vi "溶解氧电极校准.vi"() -> ()   [LabVIEW 2016, in "斯坦道多参数.lvlib"]
uses:
  <vilib>/Utility/miscctls.llb/LVPointTypeDef.ctl
  <vilib>/Analysis/NI_AALBase.lvlib
panel:
  in  "盐度自动获取":bool
  out "滤波设定":dbl
  out "标液2":string="饱和标准液"
  out "标液1":string="零点标准液"
  in  "刷新按钮":bool
  out "第二点信号值":dbl
  out "第一点信号值":dbl
  out "通讯状态":string
  out "第二点校准值":dbl
  out "第一点校准值":dbl
  out "最小值":sgl format="%#.2f"
  out "最大值":sgl format="%#.2f"
  in  "校准模式":u16(ring)=1 items=["两点校准", "单点校准"]
  in  "校准停止":bool
  in  "校准启动":bool
  out "波形图表":sgl(graph) caption="历史曲线"
  out "变异系数":dbl format="%#.6f"
  out "standard deviation":dbl caption="标准差" format="%#.2f"
  out "mean":dbl caption="均值" format="%#.2f"
  out "测量读值":dbl caption="测量值" format="%#.2f"
  out "偏移值补偿":dbl caption="溶解氧偏移修正值" format="%#.2f"
  out "饱和度值":dbl format="%#.2f"
  out "提示":string
  out "气压补偿值":dbl format="%#.2f"
  out "盐度补偿值":dbl format="%#.2f"
  out "电极斜率":dbl format="%#.6f"
  out "电极零点":dbl format="%#.6f"
  # "溶解氧电极设定"
  # "%"
  # "%"
  # "ppt"
  # "hPa"
  # "请选择校准模式:"
  # "mg/L"
  # "%"
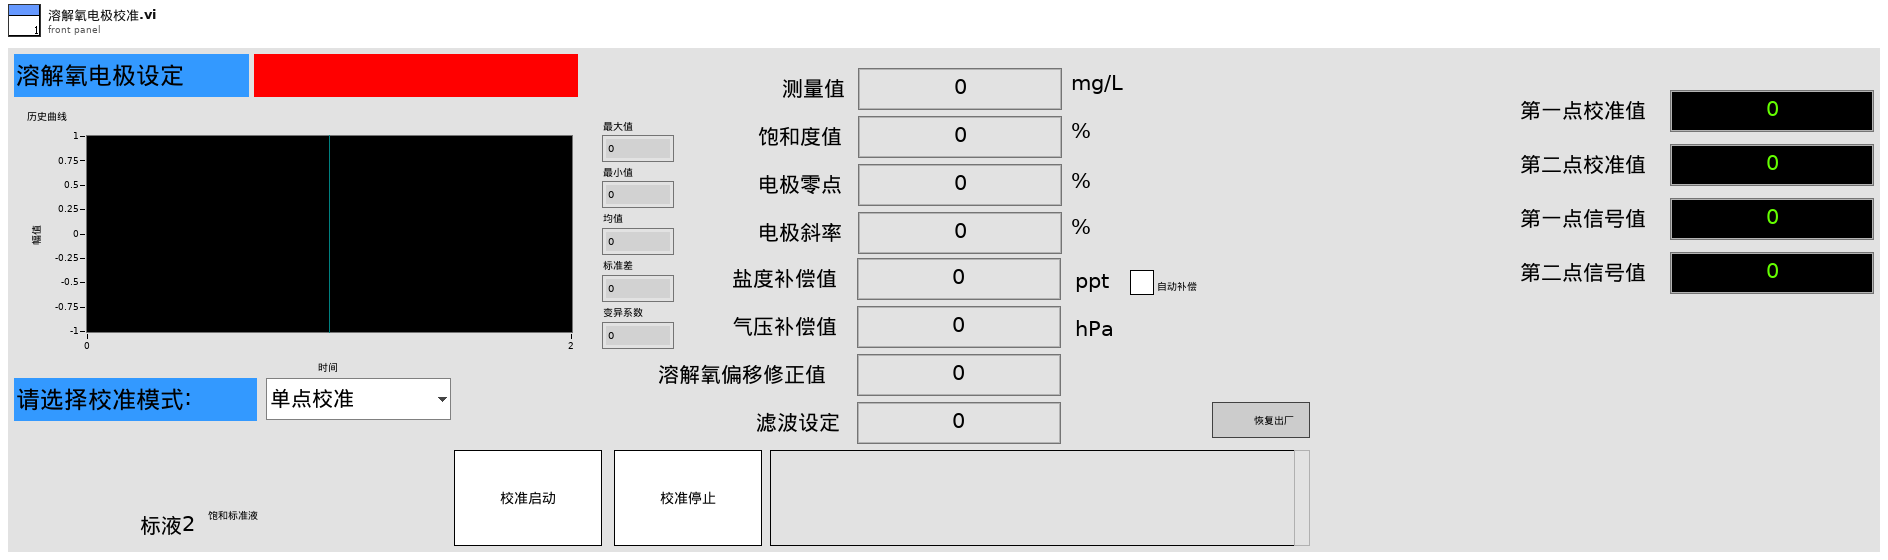
[diagram p1: front panel]
types:
  T1 = enum16{"pH", "DO", "Cond", "Turb", "ORP", "叶绿素a", "藻密度"}
  T2 = typedef "LVPointTypeDef.ctl" = cluster{"Horizontal":i16, "Vertical":i16}
  T3 = cluster{"电极状态标志":u16, "电极型号标志":u16, "溶解氧测量值":sgl, "温度测量值":sgl, "溶解氧饱和度值":sgl, "盐度补偿值":sgl, "大气压补偿值":sgl, "溶解氧偏移修正值":sgl, "温度偏移修正值":sgl, "手动温度补偿值":sgl, "溶解氧电极零点":sgl, "溶解氧电极斜率":sgl, "第1点标准值记录":sgl, "第1点信号值记录":sgl, "第1点温度值记录":sgl, "第2点标准值记录":sgl, "第2点信号值记录":sgl, "第2点温度值记录":sgl, "命令滤波设定":u16, "温度模式":enum16{"ATC", "MTC"}, "生产批次":u16, "电极序号":u16, "串口地址":u16, "串口波特率":enum16{"9600", "19200", "115200"}, "串口校验位":enum16{"NONE", "ODD", "EVEN"}, "串口停止位":enum16{"1bit", "2bit"}, "第一点标准值":sgl, "第二点标准值":sgl}
  T4 = enum8{"Enabled", "Disabled", "Disabled and Grayed Out"}
  T5 = cluster{"ph":bool, "DO":bool, "Cond":bool, "Turb":bool, "叶绿素a":bool, "藻密度":bool, "ORP":bool, "COD":bool}
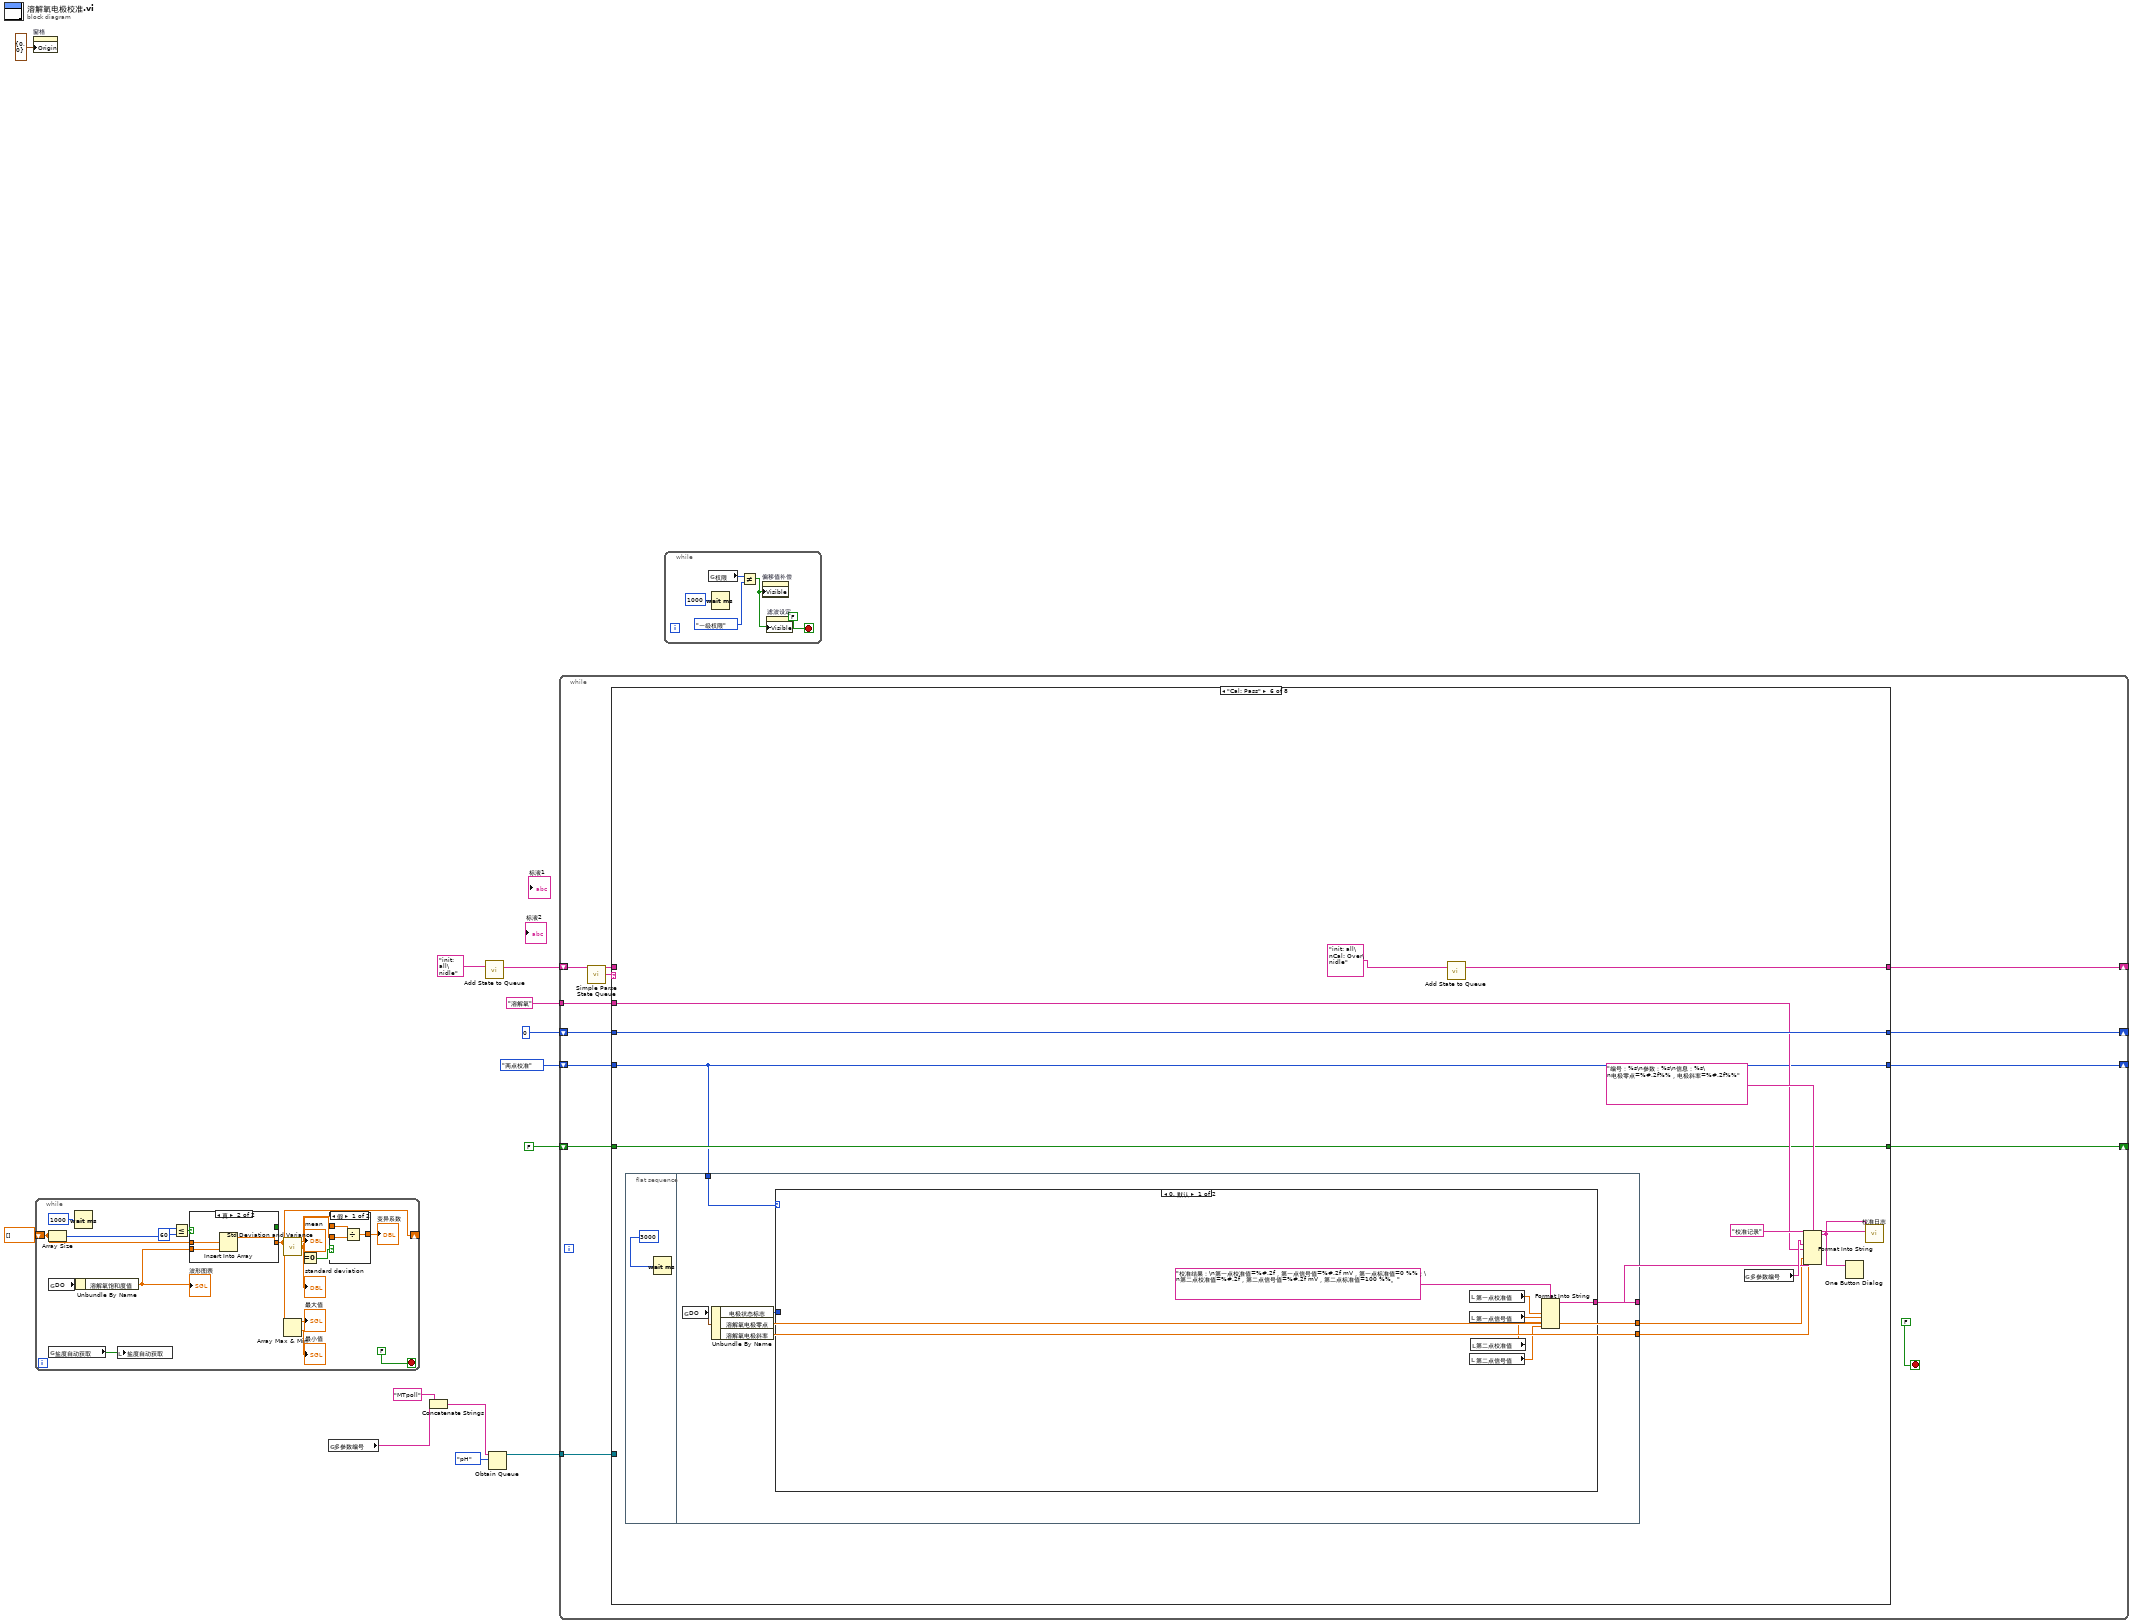
[diagram p0: block diagram]
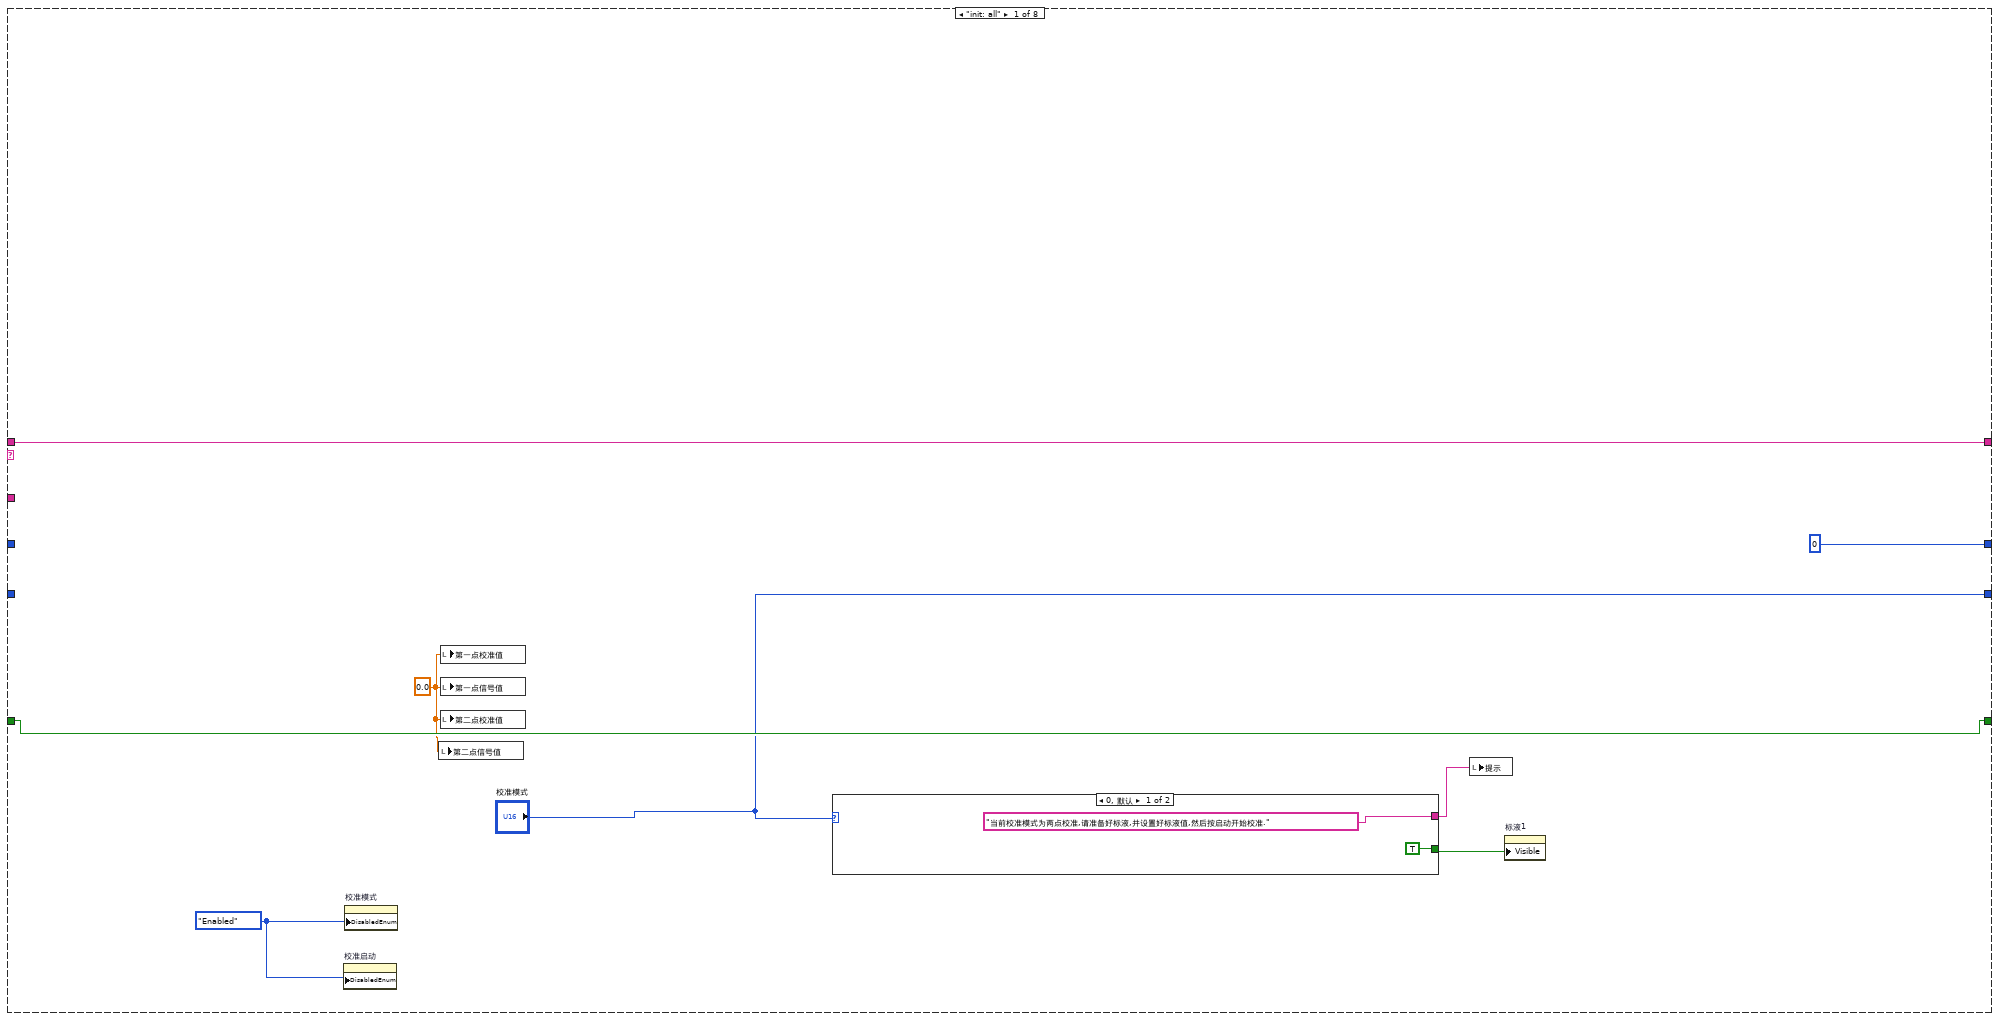
[diagram p2: hidden frame]
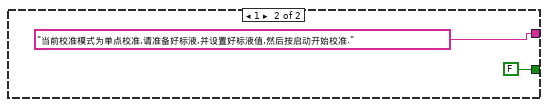
[diagram p3: hidden frame]
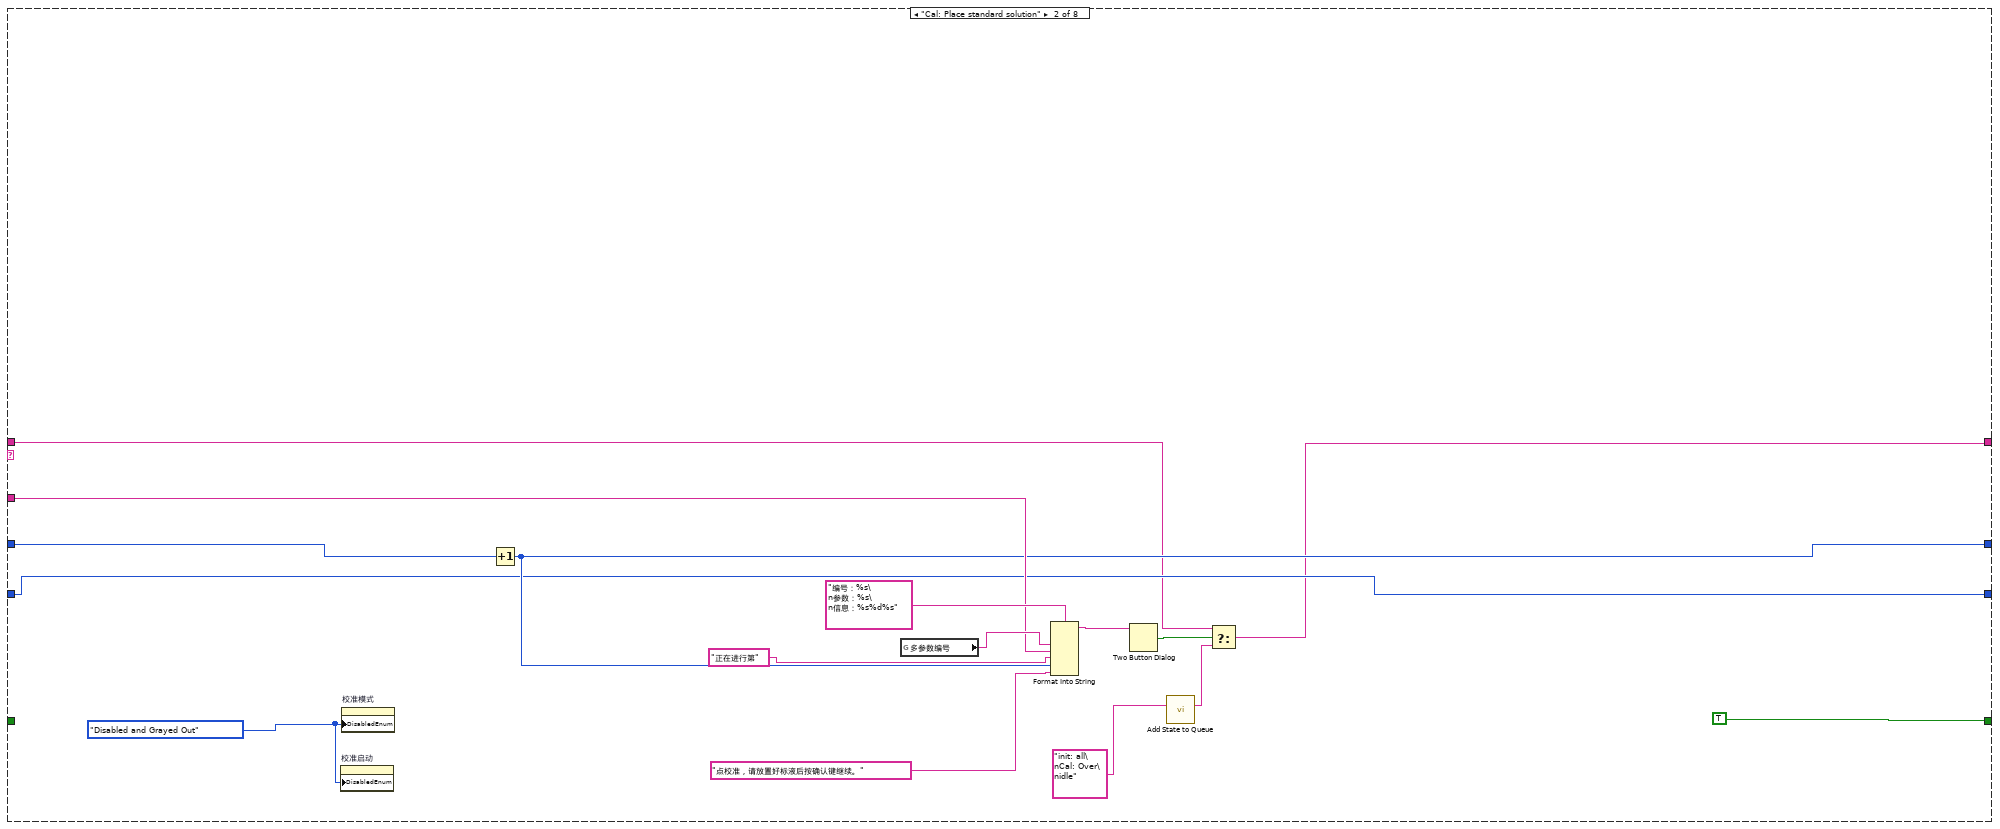
[diagram p4: hidden frame]
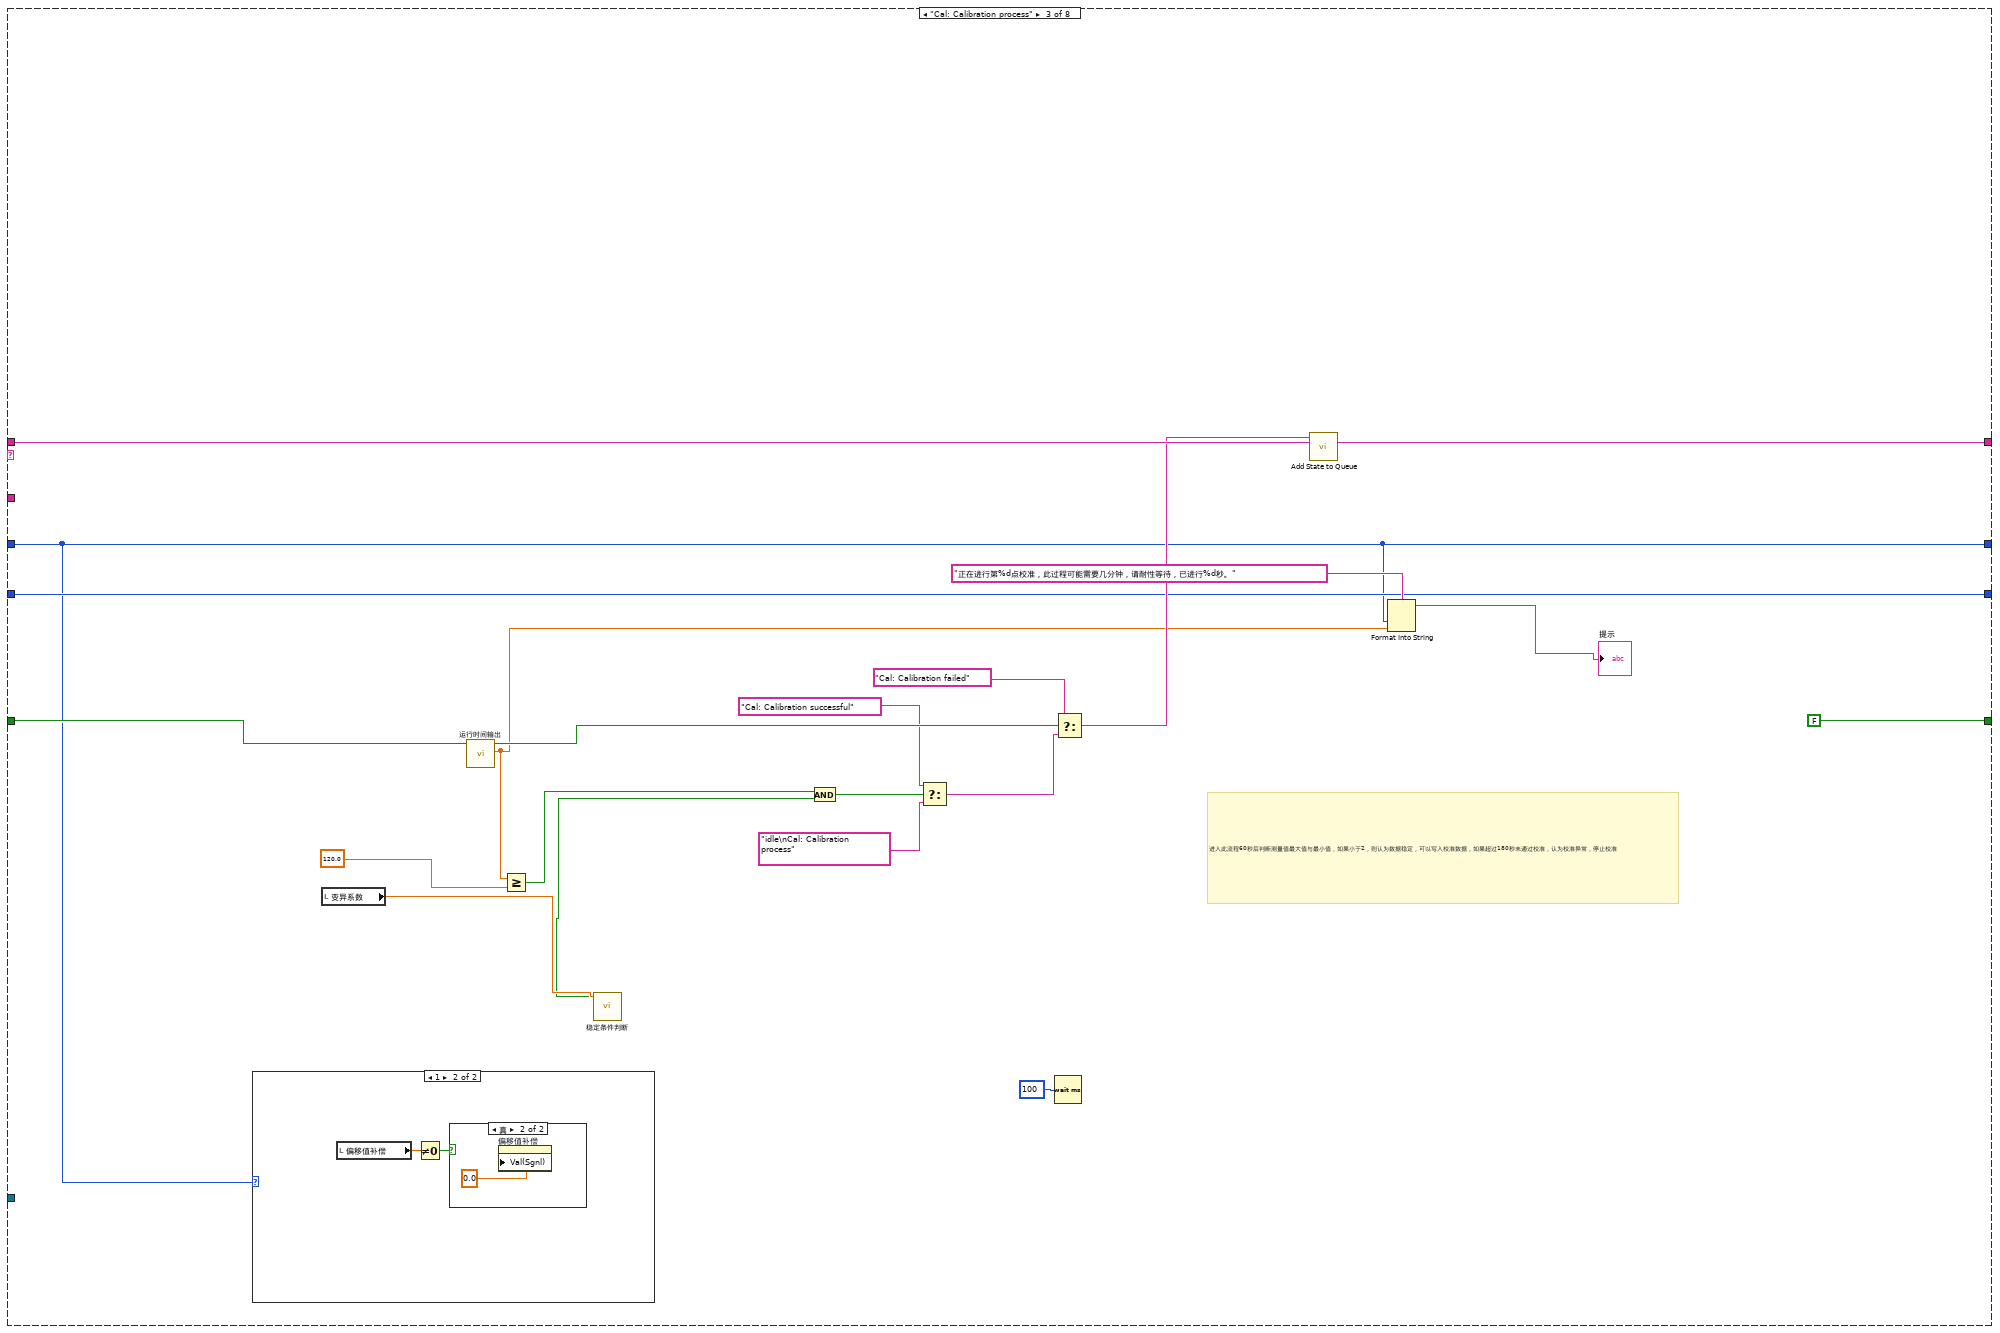
[diagram p5: hidden frame]
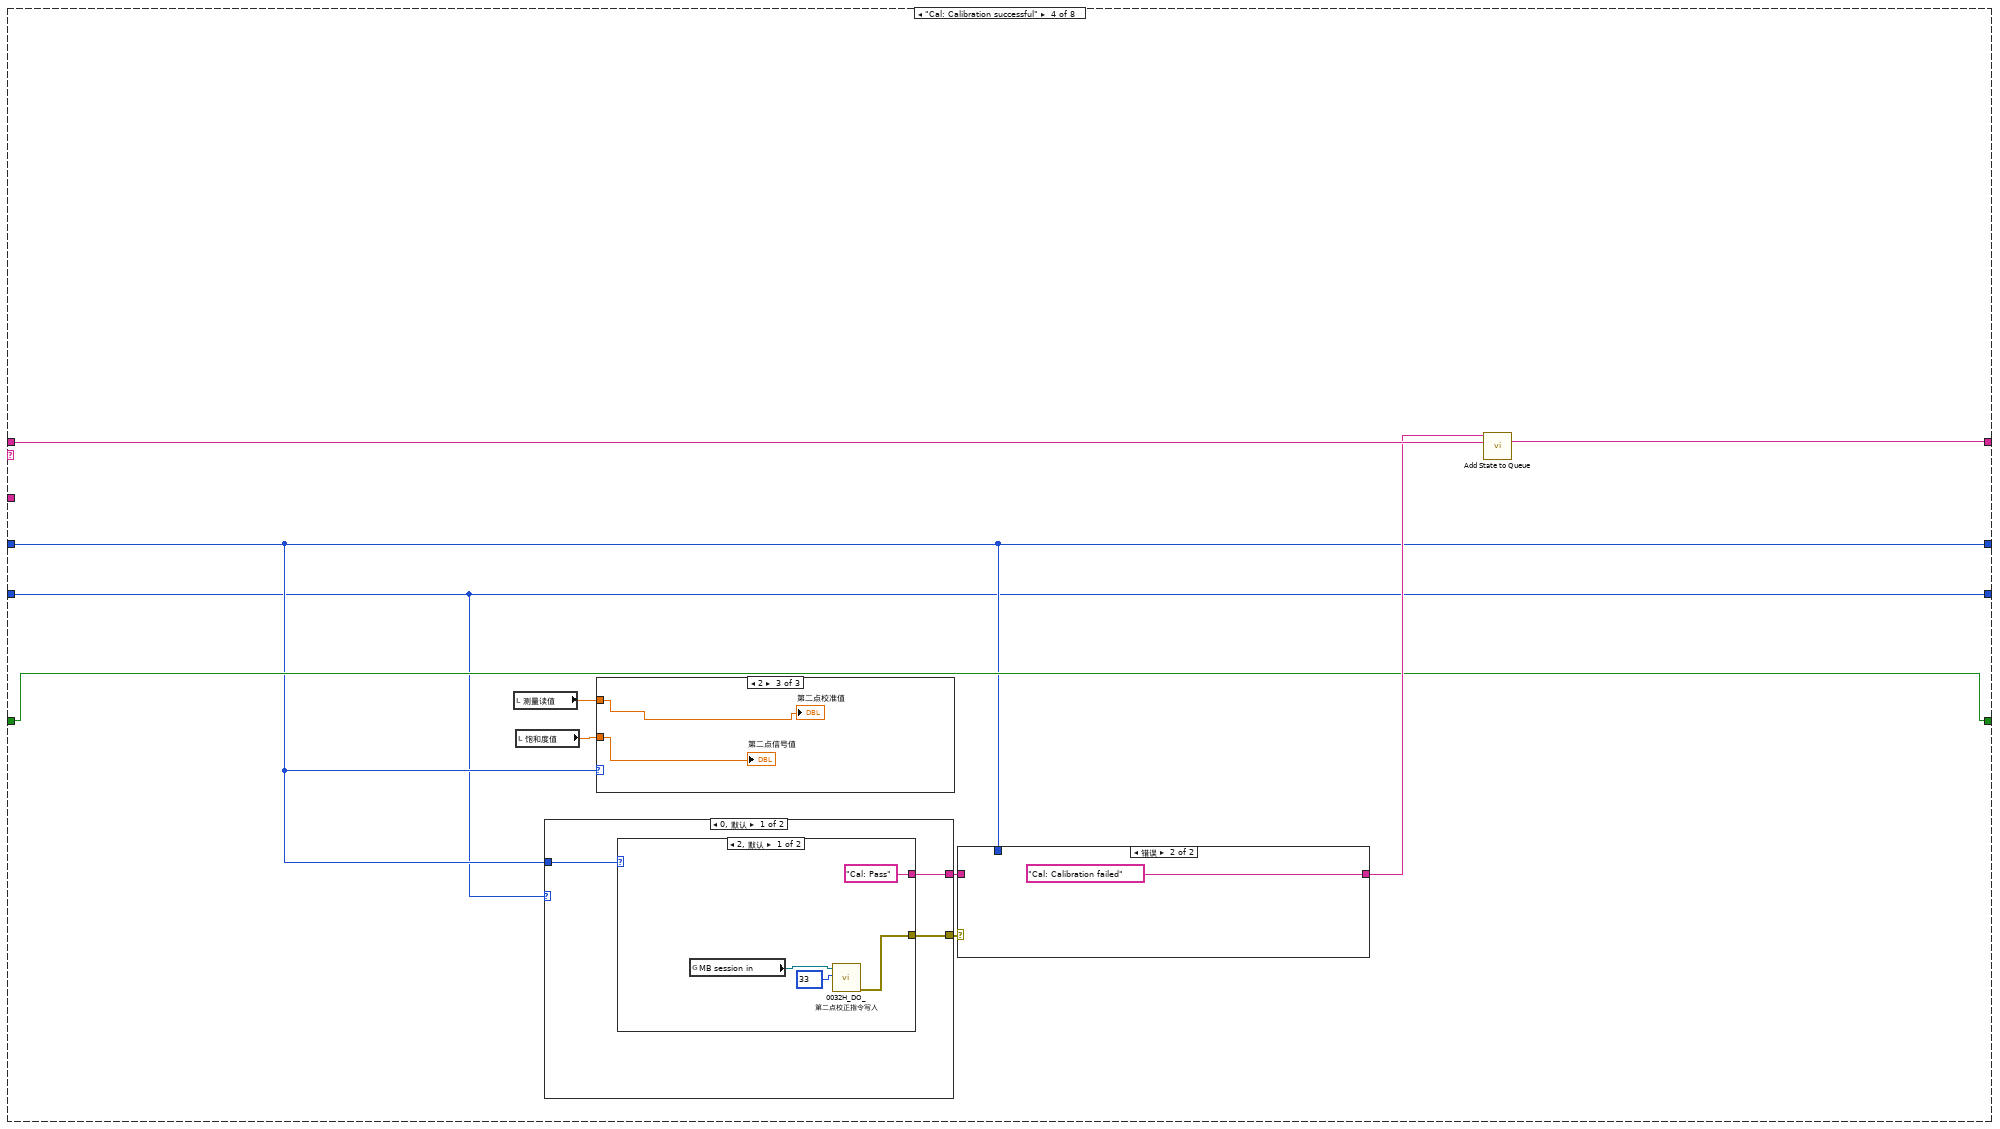
[diagram p8: hidden frame]
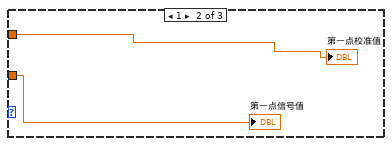
[diagram p10: hidden frame]
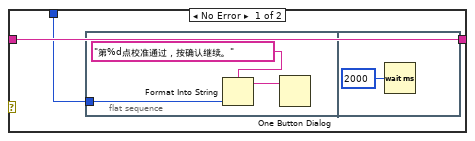
[diagram p11: hidden frame]
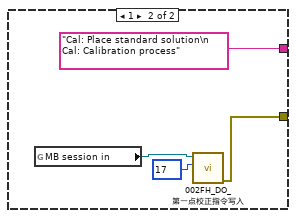
[diagram p12: hidden frame]
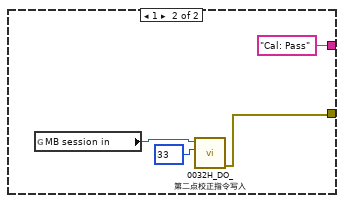
[diagram p13: hidden frame]
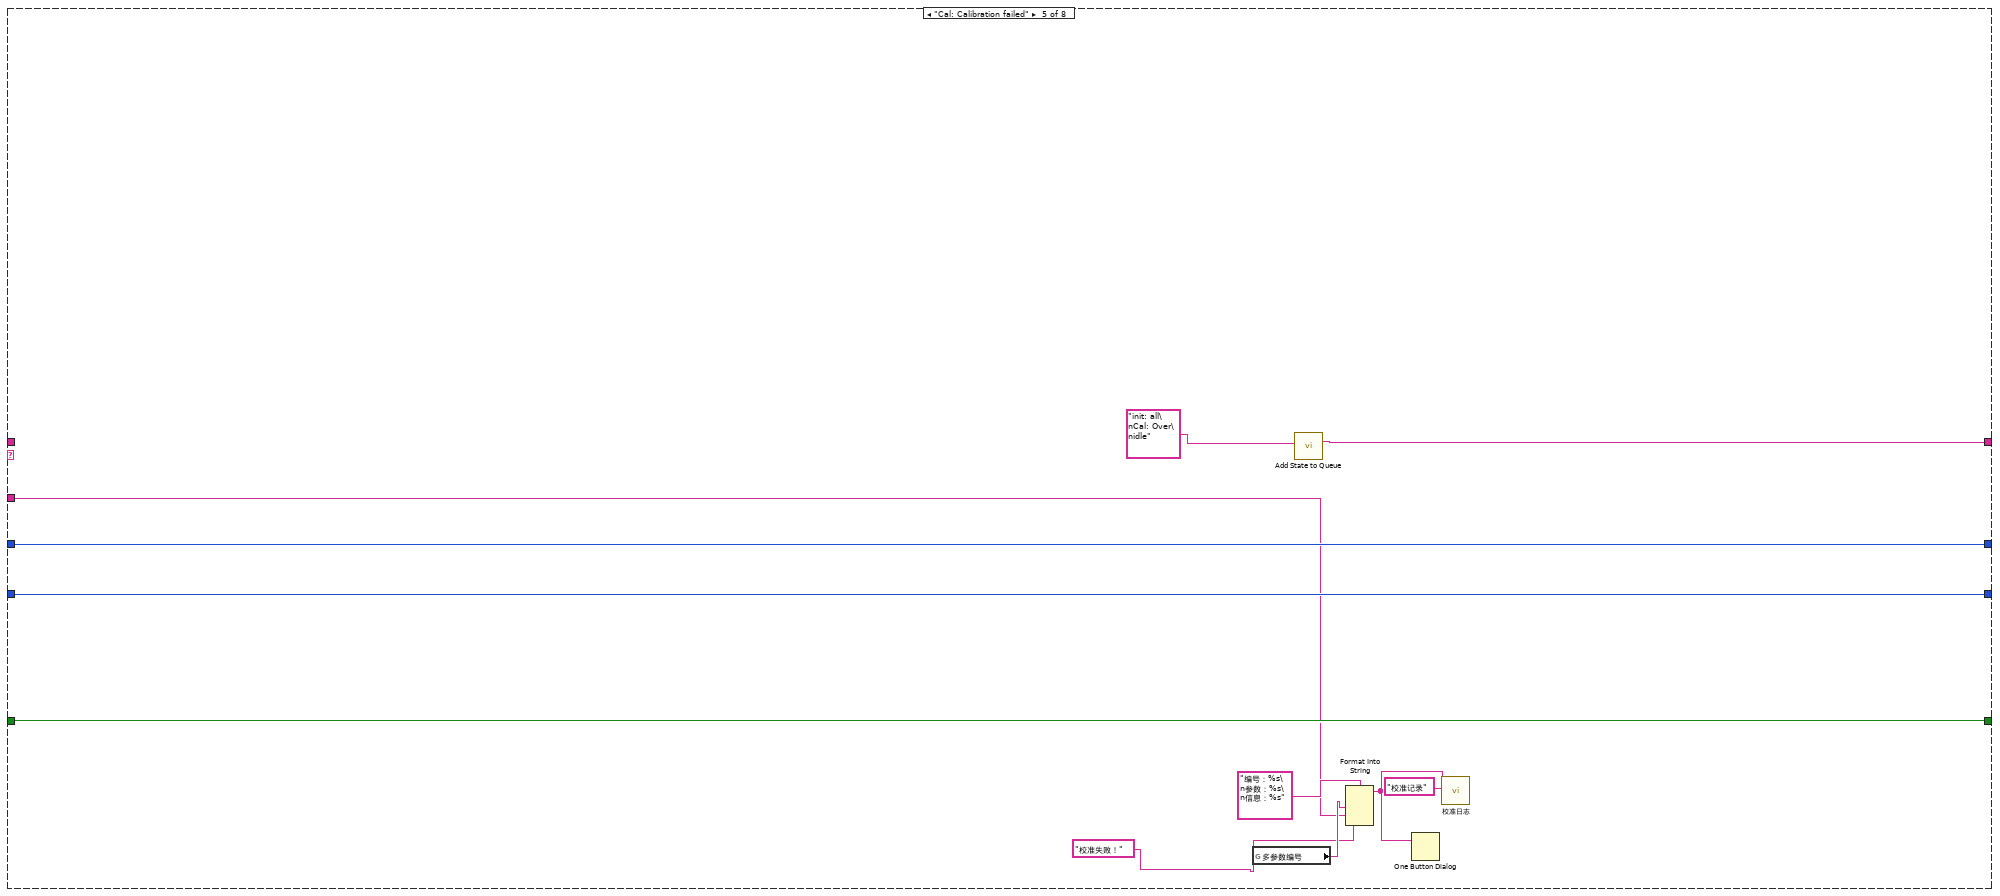
[diagram p14: hidden frame]
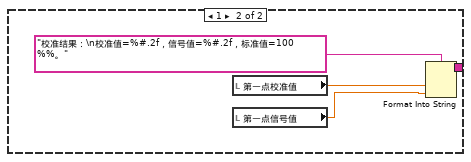
[diagram p15: hidden frame]
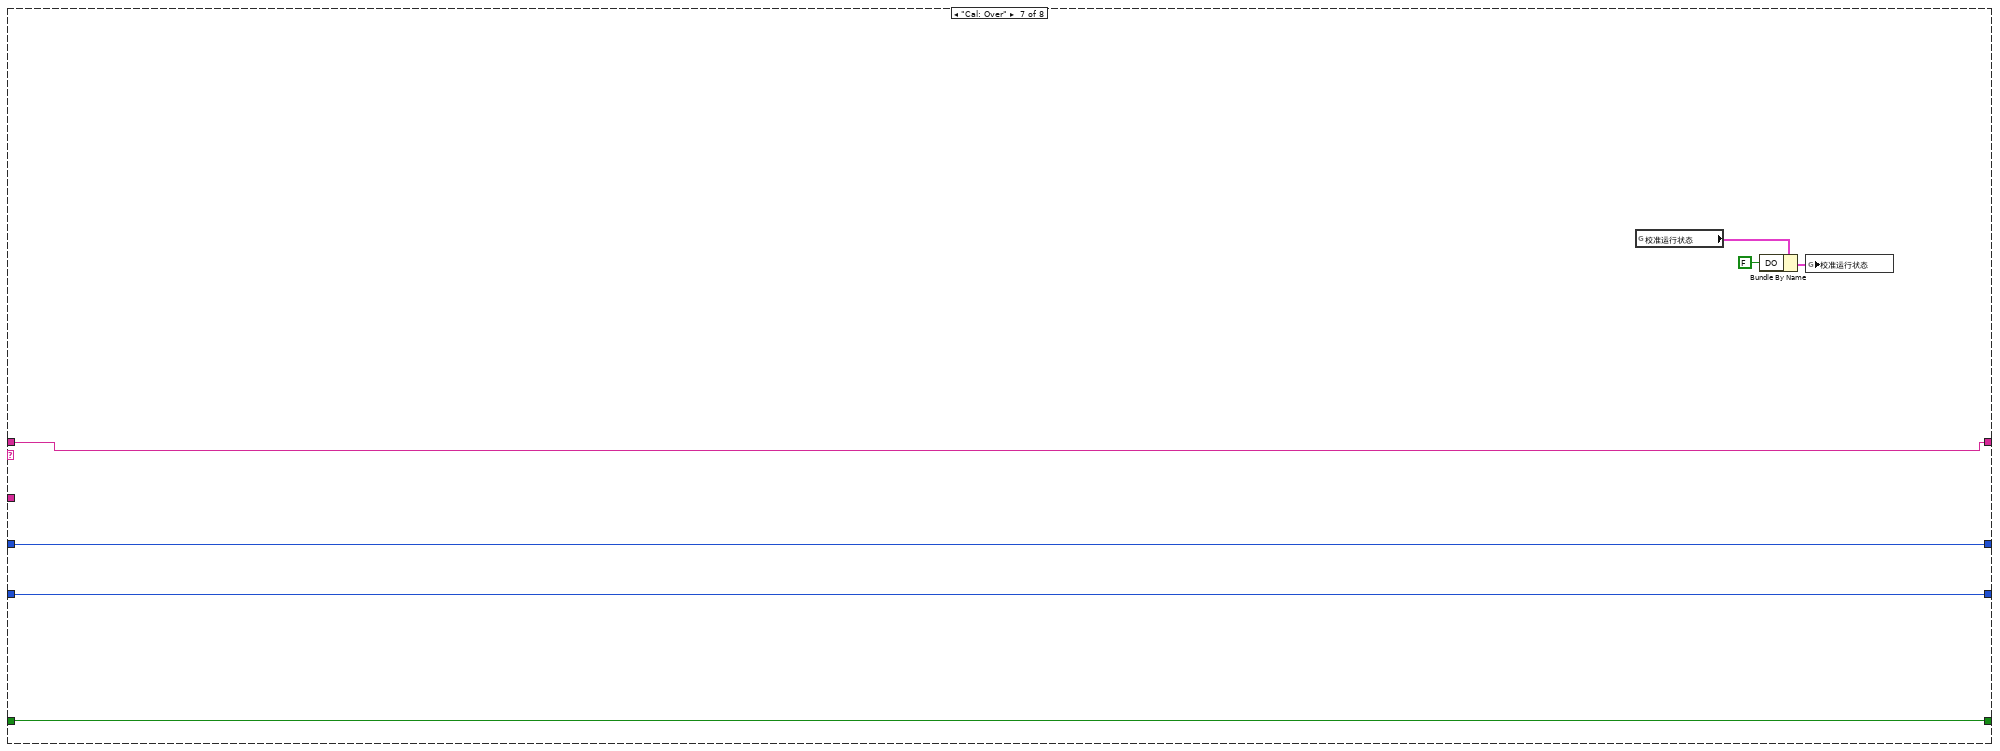
[diagram p16: hidden frame]
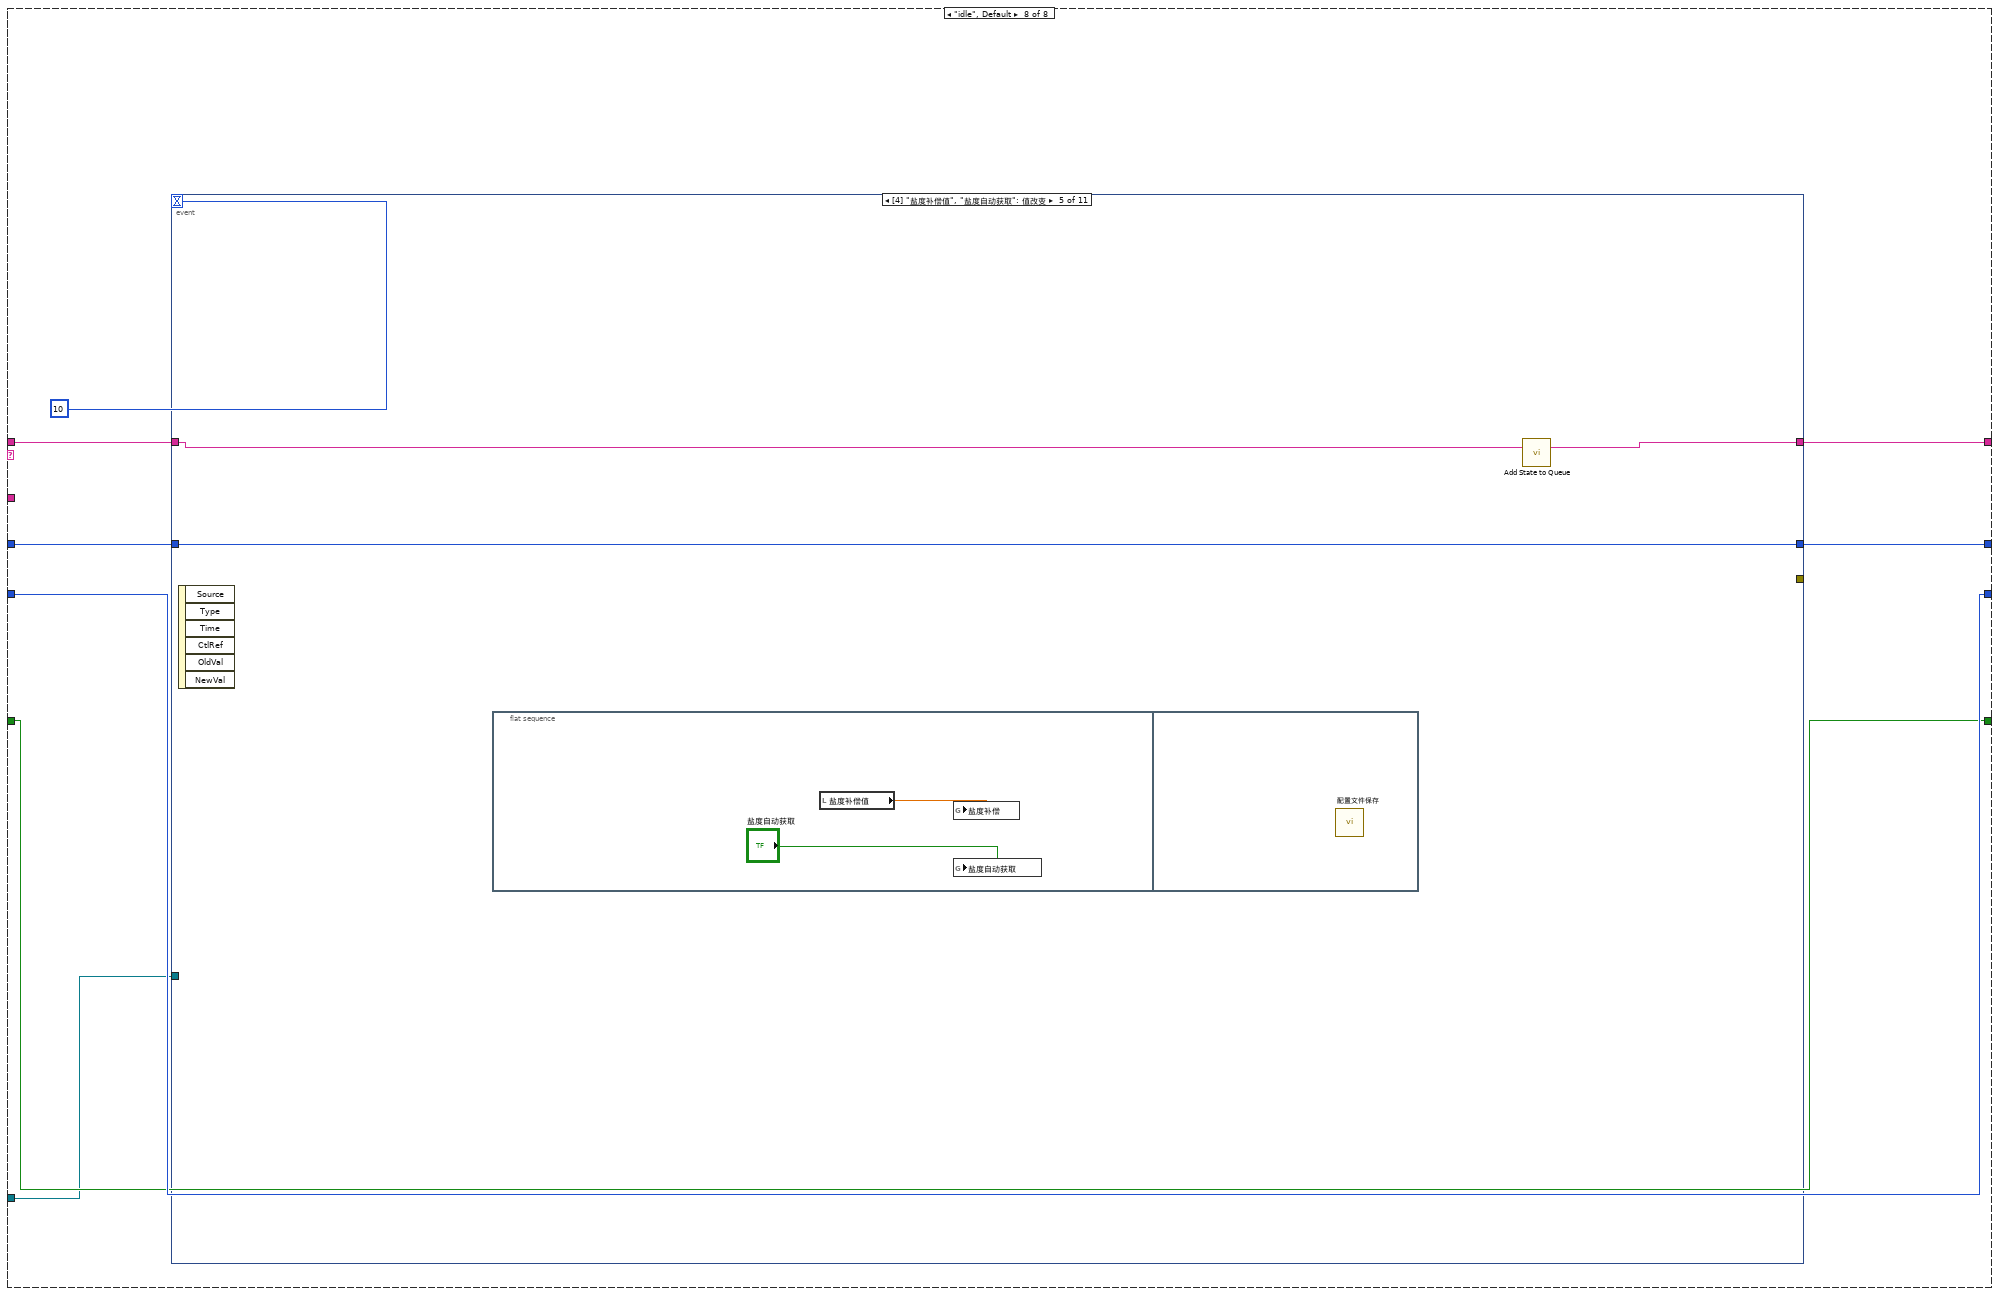
[diagram p17: hidden frame]
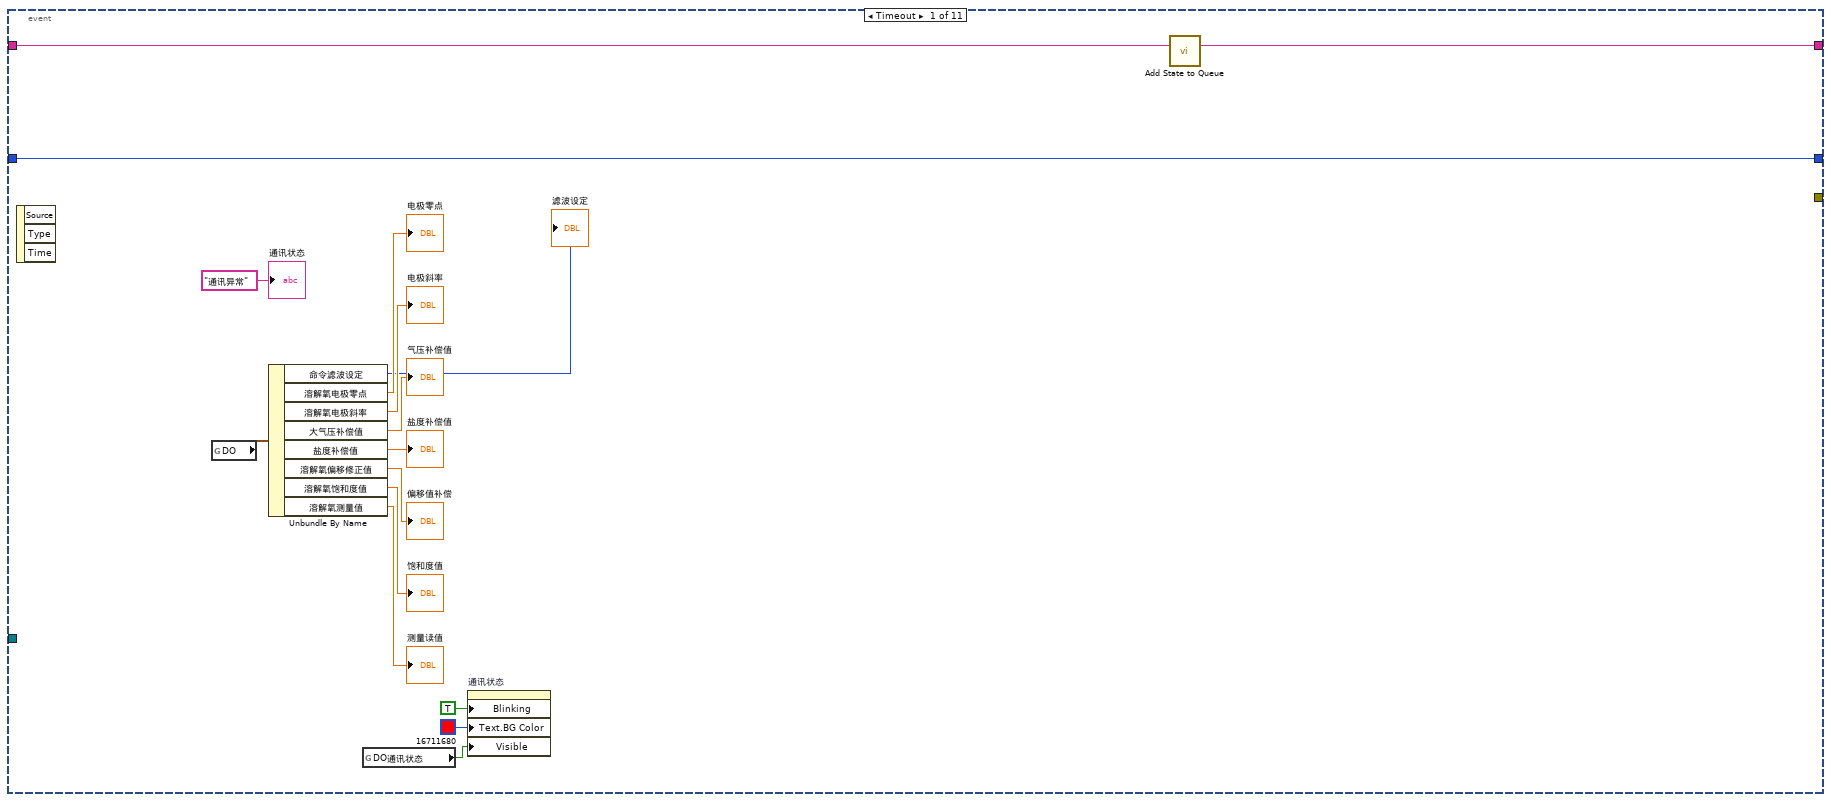
[diagram p18: hidden frame]
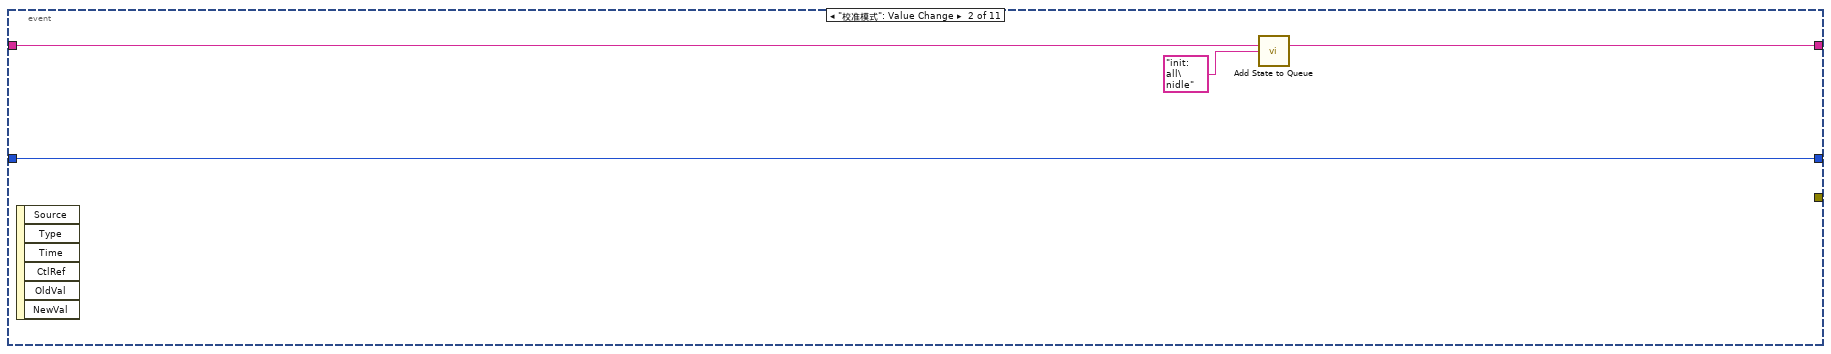
[diagram p19: hidden frame]
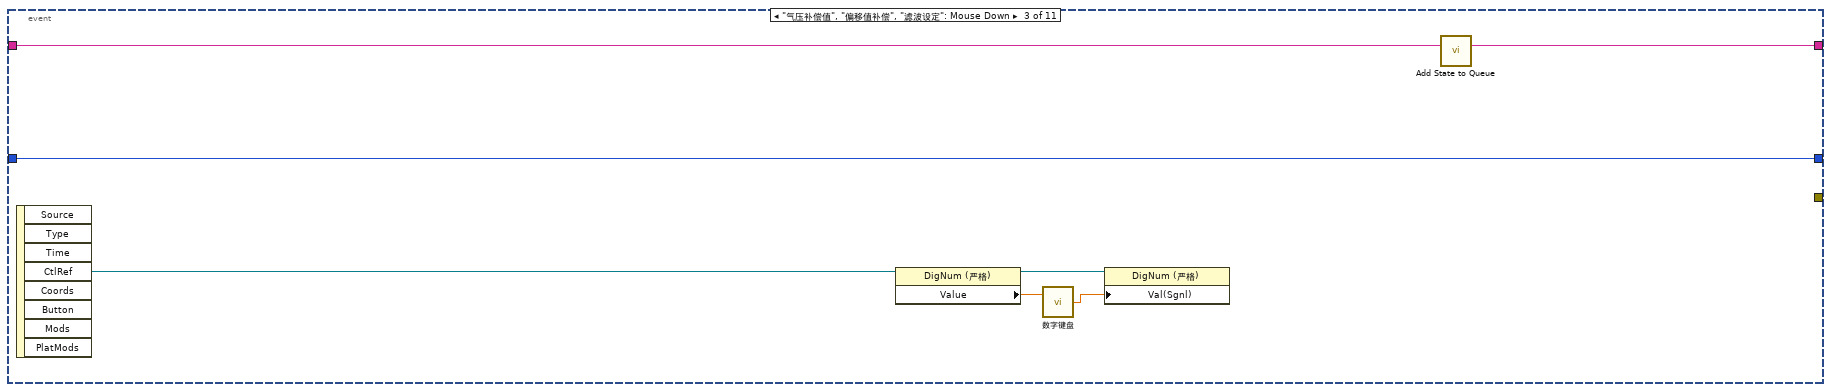
[diagram p20: hidden frame]
diagram:
  n1 = property on="窗格" class="Pane"("Origin"=T2 {"Horizontal"=0, "Vertical"=0} ("原点")) -> ()  [unwired: 2 in, 2 out]
  n2 = while {
    shift-right: [w18] -> _
    shift-left: sgl[] [] -> [w25]
    stop <- FALSE stop-if-true
    n3 = Array Size(array=w25) -> (size(s)=w27:i32)
    n4 = global read "国弘过程全局变量.vi" "DO"() -> (w21:T3)
    n5 = global read "断电保存变量.vi" "盐度自动获取"() -> (w14:bool)
    n6 = Wait (ms)(milliseconds to wait=u32 1000 ("等待时间（毫秒）")) -> ()  [unwired: 1 out]
    n7 = Unbundle By Name(w21) -> ("溶解氧饱和度值"=w15:sgl)
    "波形图表" <- w15
    n8 = local write "盐度自动获取"(w14) -> ()
    n9 = Less Or Equal?(x=w27, y=60) -> (x <= y?=w26:bool)
    n10 = case shown="真" w26 {
      tunnel: w25 -> [w38 w41]
      tunnel: w15 -> [w36 w40]
      tunnel: [w34 w39] -> w18
      tunnel: [TRUE _] -> _
      frame False {
        n11 = Replace Array Subset(array=w38, new element=w36) -> (w37:sgl[])  [unwired: 1 in]
        n12 = Rotate 1D Array(1:w37, 2:-1 ("n")) -> (0:w34:sgl[])
      }
      frame True {
        n13 = Insert Into Array(array=w41, new element=w40) -> (w39:sgl[])  [unwired: 1 in]
      }
    }
    n14 = call <vilib>:"Std Deviation and Variance.vi"("X"=w18) -> ("mean"=w20:dbl, "standard deviation"=w19:dbl)  [unwired: 1 in, 1 out]
    "mean" <- w20
    "standard deviation" <- w19
    n15 = Array Max & Min(array=w18) -> (max value=→"最大值":sgl, min value=→"最小值":sgl)  [unwired: 2 out]
    n16 = Equal To 0?(x=w20) -> (x = 0?=w24:bool)
    n17 = case shown="假" w24 {
      tunnel: w19 -> [w32 _]
      tunnel: [w31 _] -> w23
      tunnel: w20 -> [w30 _]
      frame False {
        n18 = Divide(x=w32, y=w30) -> (x/y=w31:dbl)
      }
      frame True {
      }
    }
    "变异系数" <- w23
  }
  n19 = global read "多参数全局变量.vi" "多参数编号"() -> (w2:string)
  n20 = Concatenate Strings("MTpoll" ("名称（未命名）"), w2) -> (w4:string)
  n21 = call "Add State to Queue.vi"("State(s) In (\"\")"="init: all\nidle" ("State(s) In (\"\")")) -> ("States Out"=w10:string)  [unwired: 14 in]
  n22 = Obtain Queue(name (unnamed)=w4, element data type=T1."pH" ("枚举")) -> (queue out=w1:refnum<queue>)  [unwired: 3 in, 2 out]
  n23 = while {
    shift-right: [w50] -> _
    shift-left: w10 -> [w54]
    shift-right: [w47] -> _
    shift-left: 0 -> [w49]
    tunnel: "溶解氧" ("State(s) In (\"\")") -> [w48]
    shift-right: [w45] -> _
    shift-left: enum16{"两点校准", "单点校准"}."两点校准" ("校准模式") -> [w46]
    shift-right: [w43] -> _
    shift-left: FALSE -> [w44]
    tunnel: w1 -> [w42]
    stop <- FALSE stop-if-true
    n24 = call "Simple Parse State Queue.vi"("State Queue"=w54) -> ("Remain States"=w51:string, "Next State"=w52:string)  [unwired: 13 in]
    n25 = case shown="\"Cal: Pass\"" w52 {
      tunnel: w51 -> [w62 w70 w102 w114 _ _ w190 w198]
      tunnel: [w62 w69 w101 w113 w150 w157 w190 w197] -> w50
      tunnel: w49 -> [_ w78 w87 w108 w153 w166 w189 w195]
      tunnel: w48 -> [_ w79 _ _ w144 w162 _ _]
      tunnel: [0 w76 w87 w108 w153 w166 w189 w196] -> w47
      tunnel: w46 -> [_ w75 w88 w107 w152 w158 w188 w194]
      tunnel: ["校准模式" w75 w88 w107 w152 w158 w188 w194] -> w45
      tunnel: w44 -> [w59 _ w90 w109 w151 w161 w187 w192]
      tunnel: [w59 TRUE FALSE w109 w151 w161 w187 w192] -> w43
      tunnel: w42 -> [_ _ _ _ _ _ _ w191]
      frame "init: all" {
        w57 = T4."Enabled" ("禁用")
        w58 = 0.0 ("第一点校准值")
        n26 = property on="校准启动" class="Bool"("DisabledEnum"=w57) -> ()  [unwired: 2 in, 2 out]
        n27 = property on="校准模式" class="Ring (严格)"("DisabledEnum"=w57) -> ()  [unwired: 2 in, 2 out]
        n28 = local write "第二点信号值"(w58) -> ()
        n29 = local write "第一点校准值"(w58) -> ()
        n30 = local write "第一点信号值"(w58) -> ()
        n31 = local write "第二点校准值"(w58) -> ()
        n32 = case shown="0, 默认" "校准模式" {
          tunnel: ["当前校准模式为两点校准,请准备好标液,并设置好标液值,然后按启动开始校准." ("提示") "当前校准模式为单点校准,请准备好标液,并设置好标液值,然后按启动开始校准." ("提示")] -> w61
          tunnel: [TRUE ("可见") FALSE ("可见")] -> w55
          frame 0, Default {
          }
          frame 1 {
          }
        }
        n33 = local write "提示"(w61) -> ()
        n34 = property on="标液1" class="Str"("Visible"=w55) -> ()  [unwired: 2 in, 2 out]
      }
      frame "Cal: Place standard solution" {
        w68 = T4."Disabled and Grayed Out" ("禁用")
        n35 = property on="校准启动" class="Bool"("DisabledEnum"=w68) -> ()  [unwired: 2 in, 2 out]
        n36 = property on="校准模式" class="Ring (严格)"("DisabledEnum"=w68) -> ()  [unwired: 2 in, 2 out]
        n37 = Increment(x=w78) -> (x+1=w76:i32)
        n38 = global read "多参数全局变量.vi" "多参数编号"() -> (w81:string)
        n39 = Format Into String(format string="编号：%s\n参数：%s\n信息：%s%d%s" ("格式字符串"), w81, w79, "正在进行第" ("消息"), w76, "点校准，请放置好标液后按确认键继续。" ("消息")) -> (resulting string=w73:string)  [unwired: 2 in, 1 out]
        n40 = Two Button Dialog(message=w73) -> (T button?=w72:bool)  [unwired: 2 in]
        n41 = call "Add State to Queue.vi"("State(s) In (\"\")"="init: all\nCal: Over\nidle" ("State(s) In (\"\")")) -> ("States Out"=w71:string)  [unwired: 14 in]
        n42 = Select(t=w70, s=w72, f=w71) -> (s? t:f=w69:string)
      }
      frame "Cal: Calibration process" {
        # "进入此流程60秒后判断测量值最大值与最小值，如果小于2，则认为数据稳定，可以写入校准数据，如果超过180秒未通过校准，认为校准异常，停止校准"
        n43 = case shown="1" w87 {
          frame 0, Default {
          }
          frame 1 {
            n44 = local read "偏移值补偿"() -> (w104:dbl)
            n45 = Not Equal To 0?(x=w104) -> (x != 0?=w105:bool)
            n46 = case shown="真" w105 {
              frame False {
              }
              frame True {
                n47 = property on="偏移值补偿" class="DigNum (严格)"("Val(Sgnl)"=0.0 ("值(信号)")) -> ()  [unwired: 2 in, 2 out]
              }
            }
          }
        }
        n48 = local read "变异系数"() -> (w84:dbl)
        n49 = call "运行时间输出.vi"("初始化"=w90) -> ("Elapsed Time (s)"=w86:dbl, "Time has Elapsed"=w103:bool)  [unwired: 9 in]
        n50 = Greater Or Equal?(x=w86, y=120.0) -> (x >= y?=w98:bool)
        n51 = call "稳定条件判断.vi"("变异系数"=w84) -> ("布尔"=w83:bool)  [unwired: 10 in]
        n52 = And(x=w98, y=w83) -> (x .and. y?=w95:bool)
        n53 = Select(t="Cal: Calibration successful" ("State(s) In (\"\")"), s=w95, f="idle\nCal: Calibration process" ("State(s) In (\"\")")) -> (s? t:f=w94:string)
        n54 = Wait (ms)(milliseconds to wait=u32 100 ("等待时间（毫秒）")) -> ()  [unwired: 1 out]
        n55 = Select(t="Cal: Calibration failed" ("State(s) In (\"\")"), s=w103, f=w94) -> (s? t:f=w93:string)
        n56 = call "Add State to Queue.vi"("State(s) In Front (\"\")"=w93, "State(s) In (\"\")"=w102) -> ("States Out"=w101:string)  [unwired: 13 in]
        n57 = Format Into String(format string="正在进行第%d点校准，此过程可能需要几分钟，请耐性等待，已进行%d秒。" ("格式字符串"), w87, w86) -> (resulting string=→"提示":string)  [unwired: 2 in, 1 out]
      }
      frame "Cal: Calibration successful" {
        n58 = local read "测量读值"() -> (w110:dbl)
        n59 = local read "饱和度值"() -> (w111:dbl)
        n60 = case shown="0, 默认" w107 {
          tunnel: [w130 w139] -> w116
          tunnel: [w129 "Cal: Pass" ("State(s) In (\"\")")] -> w115
          tunnel: w108 -> [w128 _]
          frame 0, Default {
            n61 = case shown="2, 默认" w128 {
              tunnel: [w131 w135] -> w130
              tunnel: ["Cal: Pass" ("State(s) In (\"\")") "Cal: Place standard solution\n Cal: Calibration process" ("State(s) In (\"\")")] -> w129
              frame 2, Default {
                n62 = global read "多参数全局变量.vi" "MB session in"() -> (w132:refnum<class "MB_Master.lvclass">)
                n63 = call "0032H_DO_第二点校正指令写入.vi"("数值"=u16 33, "MB session in"=w132) -> ("error out"=w131:errorcluster)  [unwired: 8 in, 1 out]
              }
              frame 1 {
                n64 = global read "多参数全局变量.vi" "MB session in"() -> (w136:refnum<class "MB_Master.lvclass">)
                n65 = call "002FH_DO_第一点校正指令写入.vi"("数值"=u16 17, "MB session in"=w136) -> ("error out"=w135:errorcluster)  [unwired: 8 in, 1 out]
              }
            }
          }
          frame 1 {
            n66 = global read "多参数全局变量.vi" "MB session in"() -> (w141:refnum<class "MB_Master.lvclass">)
            n67 = call "0032H_DO_第二点校正指令写入.vi"("数值"=u16 33, "MB session in"=w141) -> ("error out"=w139:errorcluster)  [unwired: 8 in, 1 out]
          }
        }
        n68 = case shown="2" w108 {
          tunnel: w111 -> [_ w118 w120]
          tunnel: w110 -> [_ w117 w119]
          frame 0, Default {
          }
          frame 1 {
            "第一点信号值" <- w118
            "第一点校准值" <- w117
          }
          frame 2 {
            "第二点信号值" <- w120
            "第二点校准值" <- w119
          }
        }
        n69 = case shown="错误" w116 {
          tunnel: w115 -> [w122 _]
          tunnel: [w122 "Cal: Calibration failed" ("State(s) In (\"\")")] -> w112
          tunnel: w108 -> [w121 _]
          frame No Error {
            n70 = flat-sequence {
              tunnel: w121 -> [w123]
              frame #0 {
                n71 = Format Into String(format string="第%d点校准通过，按确认继续。" ("格式字符串"), w123) -> (resulting string=w125:string)  [unwired: 2 in, 1 out]
                n72 = One Button Dialog(message=w125) -> ()  [unwired: 1 in, 1 out]
              }
              frame #1 {
                n73 = Wait (ms)(milliseconds to wait=u32 2000 ("等待时间（毫秒）")) -> ()  [unwired: 1 out]
              }
            }
          }
          frame Error {
          }
        }
        n74 = call "Add State to Queue.vi"("State(s) In Front (\"\")"=w112, "State(s) In (\"\")"=w114) -> ("States Out"=w113:string)  [unwired: 13 in]
      }
      frame "Cal: Calibration failed" {
        n75 = global read "多参数全局变量.vi" "多参数编号"() -> (w147:string)
        n76 = call "Add State to Queue.vi"("State(s) In (\"\")"="init: all\nCal: Over\nidle" ("State(s) In (\"\")")) -> ("States Out"=w150:string)  [unwired: 14 in]
        n77 = Format Into String(format string="编号：%s\n参数：%s\n信息：%s" ("格式字符串"), w147, w144, "校准失败！" ("消息")) -> (resulting string=w146:string)  [unwired: 2 in, 1 out]
        n78 = One Button Dialog(message=w146) -> ()  [unwired: 1 in, 1 out]
        n79 = call "校准日志.vi"("table"="校准记录", "日志信息"=w146) -> ()  [unwired: 9 in, 1 out]
      }
      frame "Cal: Pass" {
        n80 = flat-sequence {
          tunnel: [w171] -> w159
          tunnel: w158 -> [w170]
          tunnel: [w169] -> w156
          tunnel: [w168] -> w155
          frame #0 {
            n81 = Wait (ms)(milliseconds to wait=u32 3000 ("等待时间（毫秒）")) -> ()  [unwired: 1 out]
          }
          frame #1 {
            n82 = global read "国弘过程全局变量.vi" "DO"() -> (w172:T3)
            n83 = Unbundle By Name(w172) -> ("电极状态标志"=w173:u16, "溶解氧电极零点"=w169:sgl, "溶解氧电极斜率"=w168:sgl)
            n84 = case shown="0, 默认" w170 {
              tunnel: [w179 w183] -> w171
              tunnel: w173 -> [_ _]
              frame 0, Default {
                n85 = local read "第一点校准值"() -> (w177:dbl)
                n86 = local read "第一点信号值"() -> (w178:dbl)
                n87 = local read "第二点信号值"() -> (w174:dbl)
                n88 = local read "第二点校准值"() -> (w175:dbl)
                n89 = Format Into String(format string="校准结果：\n第一点校准值=%#.2f，第一点信号值=%#.2f mV，第一点标准值=0 %%；\n第二点校准值=%#.2f，第二点信号值=%#.2f mV，第二点标准值=100 %%。" ("提示"), w177, w178, w175, w174) -> (resulting string=w179:string)  [unwired: 2 in, 1 out]
              }
              frame 1 {
                n90 = local read "第一点校准值"() -> (w182:dbl)
                n91 = local read "第一点信号值"() -> (w180:dbl)
                n92 = Format Into String(format string="校准结果：\n校准值=%#.2f，信号值=%#.2f，标准值=100 %%。" ("提示"), w182, w180) -> (resulting string=w183:string)  [unwired: 2 in, 1 out]
              }
            }
          }
        }
        n93 = call "Add State to Queue.vi"("State(s) In (\"\")"="init: all\nCal: Over\nidle" ("State(s) In (\"\")")) -> ("States Out"=w157:string)  [unwired: 14 in]
        n94 = global read "多参数全局变量.vi" "多参数编号"() -> (w163:string)
        n95 = Format Into String(format string="编号：%s\n参数：%s\n信息：%s\n电极零点=%#.2f%%，电极斜率=%#.2f%%" ("格式字符串"), w163, w162, w159, w156, w155) -> (resulting string=w160:string)  [unwired: 2 in, 1 out]
        n96 = One Button Dialog(message=w160) -> ()  [unwired: 1 in, 1 out]
        n97 = call "校准日志.vi"("table"="校准记录", "日志信息"=w160) -> ()  [unwired: 9 in, 1 out]
      }
      frame "Cal: Over" {
        n98 = global read "多参数全局变量.vi" "校准运行状态"() -> (w185:T5)
        n99 = Bundle By Name(cluster=w185, "DO"=FALSE) -> (w186:T5)
        n100 = global write "多参数全局变量.vi" "校准运行状态"(w186) -> ()
      }
      frame "idle", Default {
        n101 = event shown="[4] \"盐度补偿值\", \"盐度自动获取\": 值改变" {
          selector: _ -> [_ _ _ _ _ _ _ _ _ _ _]
          dyn-events: _ -> [_ _ _ _ _ _ _ _ _ _ _]
          timeout: 10 -> [_ _ _ _ _ _ _ _ _ _ _]
          tunnel: [_ _ _ _ _ w242 w251 w260 _ _ _] -> _
          tunnel: w198 -> [w214 w218 w223 w228 w235 w246 w252 w261 w269 w280 _]
          tunnel: [w213 w217 w224 w229 w236 w247 w256 w265 w268 w279 w282] -> w197
          tunnel: [w212 w215 w225 w230 w237 w248 w257 w266 w267 w277 w283] -> w196
          tunnel: w195 -> [w212 w215 w225 w230 w237 w248 w257 w266 w267 w277 w283]
          tunnel: w191 -> [_ _ _ _ _ w241 w250 w259 _ _ _]
          event Timeout {
            n102 = event-data() -> ()  [unwired: 1 in, 3 out]
            n103 = global read "国弘过程全局变量.vi" "DO"() -> (w200:T3)
            n104 = Unbundle By Name(w200) -> ("命令滤波设定"=→"滤波设定":u16, "溶解氧电极零点"=→"电极零点":sgl, "溶解氧电极斜率"=→"电极斜率":sgl, "大气压补偿值"=→"气压补偿值":sgl, "盐度补偿值"=→"盐度补偿值":sgl, "溶解氧偏移修正值"=→"偏移值补偿":sgl, "溶解氧饱和度值"=→"饱和度值":sgl, "溶解氧测量值"=→"测量读值":sgl)
            n105 = global read "多参数全局变量.vi" "DO通讯状态"() -> (w211:bool)
            n106 = property on="通讯状态" class="Str"("Blinking"=TRUE ("闪烁"), "Text.BG Color"=u32 16711680, "Visible"=w211) -> ()  [unwired: 2 in, 2 out]
            n107 = call "Add State to Queue.vi"("State(s) In (\"\")"=w214) -> ("States Out"=w213:string)  [unwired: 14 in]
            "通讯状态" <- "通讯异常" ("当前串口")
          }
          event "校准模式": Value Change {
            n108 = event-data() -> ()  [unwired: 1 in, 6 out]
            n109 = call "Add State to Queue.vi"("State(s) In (\"\")"=w218, "State(s) At Back (\"\")"="init: all\nidle" ("State(s) In (\"\")")) -> ("States Out"=w217:string)  [unwired: 13 in]
          }
          event "气压补偿值", "偏移值补偿", "滤波设定": Mouse Down {
            n110 = event-data() -> ("CtlRef"=w222:refnum<vi>)  [unwired: 1 in, 7 out]
            n111 = property class="DigNum (严格)"(reference=w222) -> (reference out=w219:refnum<vi>, "Value"=w220:dbl)  [unwired: 1 in, 1 out]
            n112 = call "数字键盘.vi"("OldNumber"=w220) -> ("NewNumber"=w221:dbl)  [unwired: 1 in]
            n113 = property class="DigNum (严格)"(reference=w219, "Val(Sgnl)"=w221) -> ()  [unwired: 1 in, 2 out]
            n114 = call "Add State to Queue.vi"("State(s) In (\"\")"=w223) -> ("States Out"=w224:string)  [unwired: 14 in]
          }
          event "盐度补偿值": Mouse Down {
            n115 = event-data() -> ("CtlRef"=w227:refnum<vi>)  [unwired: 1 in, 7 out]
            n116 = local read "盐度自动获取"() -> (w226:bool)
            n117 = case shown="真" w226 {
              tunnel: w227 -> [_ w234]
              frame False {
              }
              frame True {
                n118 = property class="DigNum (严格)"(reference=w234) -> (reference out=w232:refnum<vi>, "Value"=w231:dbl)  [unwired: 1 in, 1 out]
                n119 = call "数字键盘.vi"("显示样式"=w231) -> ("NewNumber"=w233:dbl)  [unwired: 1 in]
                n120 = property class="DigNum (严格)"(reference=w232, "Val(Sgnl)"=w233) -> ()  [unwired: 1 in, 2 out]
              }
            }
            n121 = call "Add State to Queue.vi"("State(s) In (\"\")"=w228) -> ("States Out"=w229:string)  [unwired: 14 in]
          }
          event "盐度补偿值", "盐度自动获取": Value Change {
            n122 = event-data() -> ()  [unwired: 1 in, 6 out]
            n123 = flat-sequence {
              frame #0 {
                n124 = local read "盐度补偿值"() -> (w238:dbl)
                n125 = global write "断电保存变量.vi" "盐度补偿"(w238) -> ()
                n126 = global write "断电保存变量.vi" "盐度自动获取"("盐度自动获取") -> ()
              }
              frame #1 {
                n127 = call "配置文件保存.vi"() -> ()  [unwired: 12 in]
              }
            }
            n128 = call "Add State to Queue.vi"("State(s) In (\"\")"=w235) -> ("States Out"=w236:string)  [unwired: 14 in]
          }
          event "滤波设定": Value Change {
            n129 = event-data() -> ("NewVal"=w244:dbl)  [unwired: 1 in, 5 out]
            n130 = global read "多参数全局变量.vi" "MB session in"() -> (w245:refnum<class "MB_Master.lvclass">)
            n131 = call "0027H_DO_数位滤波设定写入.vi"("数值"=w244, "MB session in"=w245) -> ("error out"=w243:errorcluster)  [unwired: 8 in, 1 out]
            n132 = Enqueue Element At Opposite End(queue=w241, element=T1."DO" ("元素"), error in (no error)=w243) -> (error out=w242:errorcluster)  [unwired: 1 in, 2 out]
            n133 = call "Add State to Queue.vi"("State(s) In (\"\")"=w246) -> ("States Out"=w247:string)  [unwired: 14 in]
          }
          event "气压补偿值": Value Change {
            n134 = event-data() -> ("NewVal"=w254:dbl)  [unwired: 1 in, 5 out]
            n135 = global read "多参数全局变量.vi" "MB session in"() -> (w255:refnum<class "MB_Master.lvclass">)
            n136 = call "000AH_DO_大气压补偿值写入.vi"("数值"=w254, "MB session in"=w255) -> ("error out"=w253:errorcluster)  [unwired: 8 in, 1 out]
            n137 = Enqueue Element At Opposite End(queue=w250, element=T1."DO" ("元素"), error in (no error)=w253) -> (error out=w251:errorcluster)  [unwired: 1 in, 2 out]
            n138 = call "Add State to Queue.vi"("State(s) In (\"\")"=w252) -> ("States Out"=w256:string)  [unwired: 14 in]
          }
          event "偏移值补偿": Value Change {
            n139 = event-data() -> ("NewVal"=w263:dbl)  [unwired: 1 in, 5 out]
            n140 = global read "多参数全局变量.vi" "MB session in"() -> (w264:refnum<class "MB_Master.lvclass">)
            n141 = call "000CH_DO_DO偏移修正值写入.vi"("数值"=w263, "MB session in"=w264) -> ("error out"=w262:errorcluster)  [unwired: 8 in, 1 out]
            n142 = Enqueue Element At Opposite End(queue=w259, element=T1."DO" ("元素"), error in (no error)=w262) -> (error out=w260:errorcluster)  [unwired: 1 in, 2 out]
            n143 = call "Add State to Queue.vi"("State(s) In (\"\")"=w261) -> ("States Out"=w265:string)  [unwired: 14 in]
          }
          event "刷新按钮": Value Change {
            n144 = event-data() -> ()  [unwired: 1 in, 6 out]
            n145 = call "Add State to Queue.vi"("State(s) In (\"\")"=w269) -> ("States Out"=w268:string)  [unwired: 14 in]
            n146 = Two Button Dialog(message="请再次确实是否恢复出厂设置！" ("消息")) -> (T button?=w271:bool)  [unwired: 2 in]
            n147 = case shown="真" w271 {
              frame False {
              }
              frame True {
                w272 = u16 33 items=["Factory Reset"=33] ("数值")
                n148 = global read "多参数全局变量.vi" "MB session in"() -> (w273:refnum<class "MB_Master.lvclass">)
                n149 = call "0026H_DO_命令寄存器写入.vi"("数值"=w272, "MB session in"=w273) -> ()  [unwired: 8 in, 2 out]
              }
            }
          }
          event "校准启动": Value Change {
            n150 = event-data() -> ()  [unwired: 1 in, 6 out]
            n151 = global read "多参数全局变量.vi" "校准运行状态"() -> (w275:T5)
            n152 = call "Add State to Queue.vi"("State(s) In (\"\")"=w280, "State(s) At Back (\"\")"="init: all\nCal: Place standard solution\n Cal: Calibration process\nidle" ("State(s) In (\"\")")) -> ("States Out"=w279:string)  [unwired: 13 in]
            n153 = Bundle By Name(cluster=w275, "DO"=TRUE) -> (w276:T5)
            n154 = global write "多参数全局变量.vi" "校准运行状态"(w276) -> ()
          }
          event "校准停止": Value Change {
            n155 = event-data() -> ()  [unwired: 1 in, 6 out]
            n156 = call "Add State to Queue.vi"("State(s) In (\"\")"="init: all\nCal: Over\nidle" ("State(s) In (\"\")")) -> ("States Out"=w282:string)  [unwired: 14 in]
          }
        }
      }
    }
  }
  n157 = while {
    stop <- FALSE stop-if-true
    n158 = global read "多参数全局变量.vi" "权限"() -> (w287:enum16{"一级权限", "二级权限", "三级权限"})
    n159 = Wait (ms)(milliseconds to wait=u32 1000 ("等待时间（毫秒）")) -> ()  [unwired: 1 out]
    n160 = Not Equal?(x=w287, y=enum16{"一级权限", "二级权限", "三级权限"}."一级权限") -> (x != y?=w284:bool)
    n161 = property on="偏移值补偿" class="DigNum (严格)"("Visible"=w284) -> ()  [unwired: 2 in, 2 out]
    n162 = property on="滤波设定" class="DigNum (严格)"("Visible"=w284) -> ()  [unwired: 2 in, 2 out]
  }
